vi "(Test) Chamber.vi"() -> ()   [LabVIEW 2017]
uses:
  f30135b8-ed91-49ac-be03-38adf51057fc.vi
  a24e3ecb-3937-427e-89a7-e138db600c34.vi
  c2173d89-5ae8-4599-a943-d35810f265fc.vi
  2c7cd04d-549a-457e-88ac-024da1df5a93.vi
  <vilib>/Instr/_visa.llb/VISA Configure Serial Port (Instr).vi
panel:
  out "*(타입 *) &x":string
  in  "Taget Temp":u16
  out "Data":string
  out "Write":string
  out "CRC16":string
  out "READ":string
  # "15"
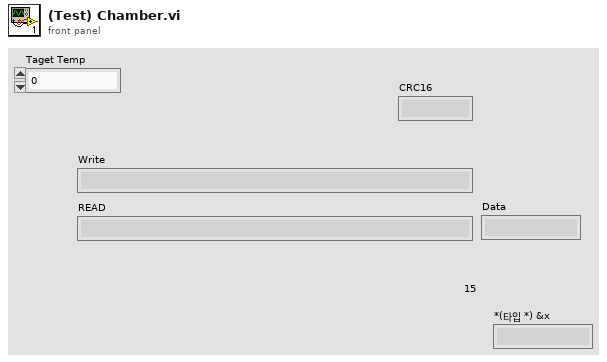
[diagram p1: front panel]
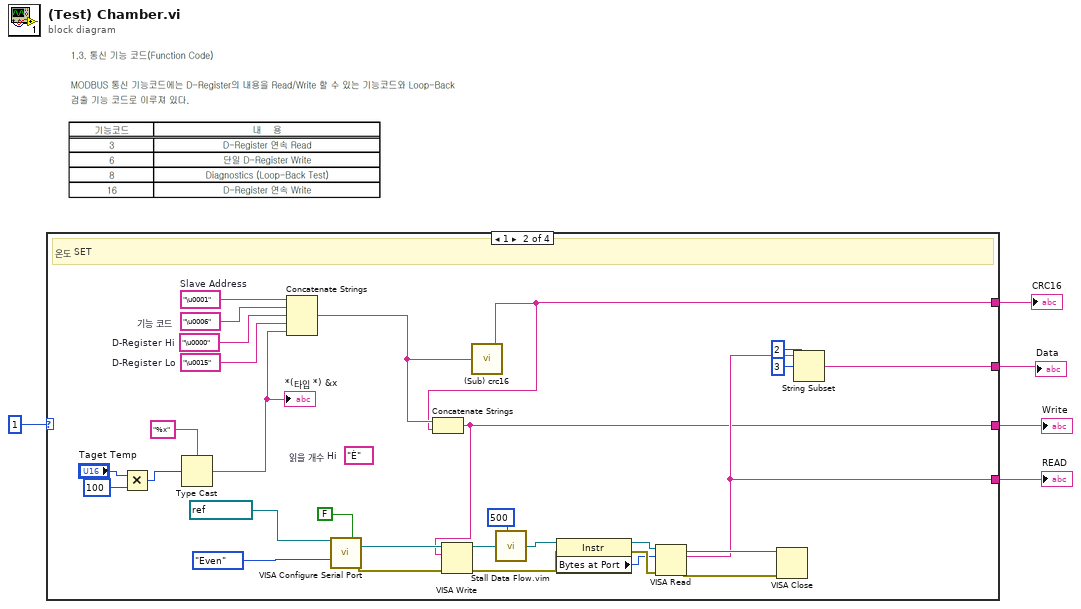
[diagram p0: block diagram]
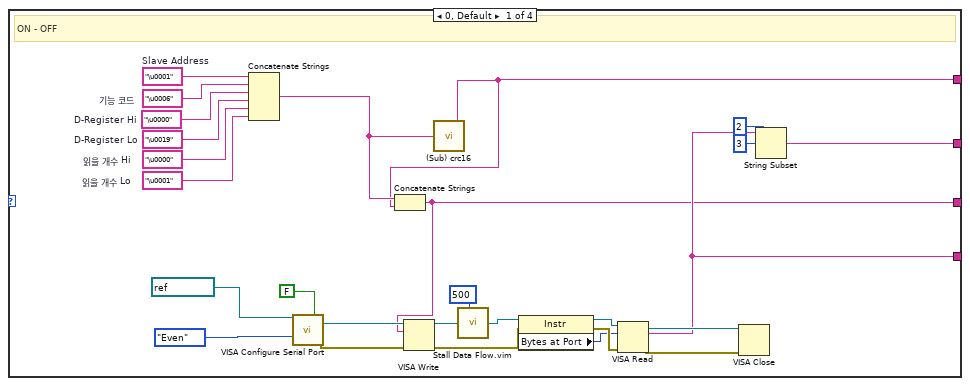
[diagram p2: hidden frame]
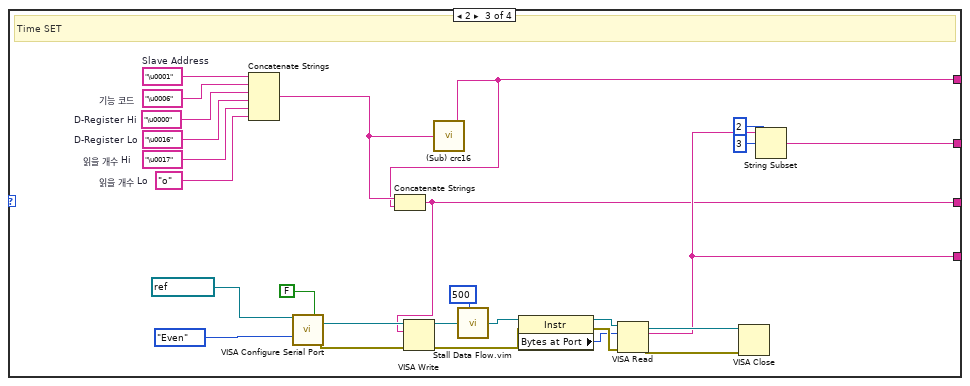
[diagram p3: hidden frame]
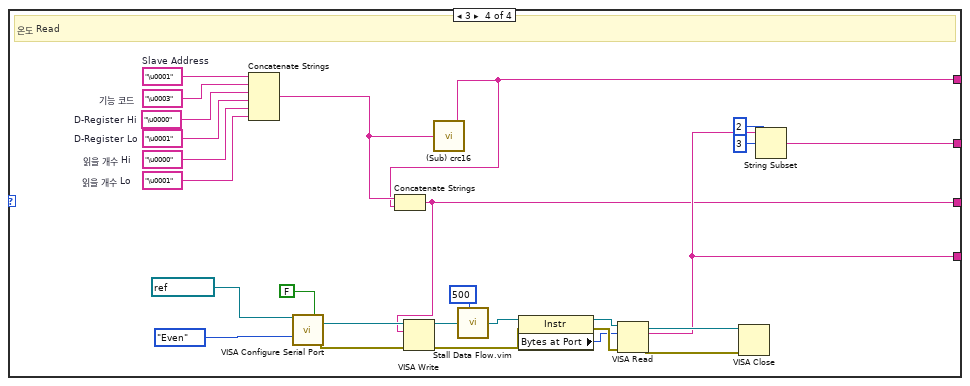
[diagram p4: hidden frame]
diagram:
  n1 = case shown="1" 1 {
    tunnel: [w9 w41 w66 w93] -> w5
    tunnel: [w8 w40 w65 w92] -> w4
    tunnel: [w7 w39 w64 w91] -> w3
    tunnel: [w6 w38 w63 w90] -> w2
    frame 0, Default {
      w10 = "\u0001"  # 읽을 개수 Lo
      w16 = "\u0000"  # 읽을 개수 Hi
      w17 = "\u0019"  # D-Register Lo
      w18 = "\u0000"  # D-Register Hi
      w19 = "\u0006"  # 기능 코드
      w20 = "\u0001"  # Slave Address
      # "ON - OFF"
      n2 = Concatenate Strings(w20, w19, w18, w17, w16, w10) -> (w15:string)
      n3 = call-poly "VISA Configure Serial Port"("VISA resource name"=refnum<visa-resource-name> "COM7", "Enable Termination\nChar (T)"=FALSE ("Enable Termination\nChar (T)"), "parity (0:none)"=enum16{"None", "Odd", "Even", "Mark", "Space"}."Even") -> ("VISA resource name out"=w32:refnum<visa-resource-name>, "error out"=w31:errorcluster)  [unwired: 11 in]
      n4 = call "(Sub) crc16.vi"("message"=w15) -> ("CRC16"=w9:string)  [unwired: 4 in]
      n5 = Concatenate Strings(w15, w9) -> (w6:string)
      n6 = VISA Write(VISA resource name=w32, write buffer=w6, error in (no error)=w31) -> (VISA resource name out=w28:refnum<visa-resource-name>, error out=w27:errorcluster)  [unwired: 1 out]
      n7 = call "Stall Data Flow.vim"("value in"=w28, "milliseconds to wait"=u32 500) -> ("value out"=w22:refnum<visa-resource-name>)  [unwired: 1 out]
      n8 = property class="Instr"(reference=w22, error in=w27) -> (reference out=w26:refnum<visa-resource-name>, error out=w25:errorcluster, "Bytes at Port"=w14:u32)
      n9 = VISA Read(VISA resource name=w26, byte count=w14, error in (no error)=w25) -> (VISA resource name out=w30:refnum<visa-resource-name>, read buffer=w7:string, error out=w29:errorcluster)  [unwired: 1 out]
      n10 = VISA Close(VISA resource name=w30, error in (no error)=w29) -> ()  [unwired: 1 out]
      n11 = String Subset(string=w7, offset (0)=3 ("오프셋(0)"), length (rest)=2 ("길이(나머지)")) -> (substring=w8:string)
    }
    frame 1 {
      (unwired) "È"  # 읽을 개수 Hi
      w47 = "\u0015"  # D-Register Lo
      w48 = "\u0000"  # D-Register Hi
      w49 = "\u0006"  # 기능 코드
      w50 = "\u0001"  # Slave Address
      # "온도 SET"
      n12 = Multiply(x="Taget Temp", y=u16 100) -> (x*y=w33:u16)
      n13 = Type Cast(type="%x" ("타입"), x=w33) -> (*(type *) &x=w36:string)
      "*(타입 *) &x" <- w36
      n14 = Concatenate Strings(w50, w49, w48, w47, w36) -> (w46:string)
      n15 = call-poly "VISA Configure Serial Port"("VISA resource name"=refnum<visa-resource-name> "COM7", "Enable Termination\nChar (T)"=FALSE ("Enable Termination\nChar (T)"), "parity (0:none)"=enum16{"None", "Odd", "Even", "Mark", "Space"}."Even") -> ("VISA resource name out"=w62:refnum<visa-resource-name>, "error out"=w61:errorcluster)  [unwired: 11 in]
      n16 = call "(Sub) crc16.vi"("message"=w46) -> ("CRC16"=w41:string)  [unwired: 4 in]
      n17 = Concatenate Strings(w46, w41) -> (w38:string)
      n18 = VISA Write(VISA resource name=w62, write buffer=w38, error in (no error)=w61) -> (VISA resource name out=w58:refnum<visa-resource-name>, error out=w57:errorcluster)  [unwired: 1 out]
      n19 = call "Stall Data Flow.vim"("value in"=w58, "milliseconds to wait"=u32 500) -> ("value out"=w52:refnum<visa-resource-name>)  [unwired: 1 out]
      n20 = property class="Instr"(reference=w52, error in=w57) -> (reference out=w56:refnum<visa-resource-name>, error out=w55:errorcluster, "Bytes at Port"=w45:u32)
      n21 = VISA Read(VISA resource name=w56, byte count=w45, error in (no error)=w55) -> (VISA resource name out=w60:refnum<visa-resource-name>, read buffer=w39:string, error out=w59:errorcluster)  [unwired: 1 out]
      n22 = VISA Close(VISA resource name=w60, error in (no error)=w59) -> ()  [unwired: 1 out]
      n23 = String Subset(string=w39, offset (0)=3 ("오프셋(0)"), length (rest)=2 ("길이(나머지)")) -> (substring=w40:string)
    }
    frame 2 {
      w67 = "o"  # 읽을 개수 Lo
      w73 = "\u0017"  # 읽을 개수 Hi
      w74 = "\u0016"  # D-Register Lo
      w75 = "\u0000"  # D-Register Hi
      w76 = "\u0006"  # 기능 코드
      w77 = "\u0001"  # Slave Address
      # "Time SET"
      n24 = Concatenate Strings(w77, w76, w75, w74, w73, w67) -> (w72:string)
      n25 = call-poly "VISA Configure Serial Port"("VISA resource name"=refnum<visa-resource-name> "COM7", "Enable Termination\nChar (T)"=FALSE ("Enable Termination\nChar (T)"), "parity (0:none)"=enum16{"None", "Odd", "Even", "Mark", "Space"}."Even") -> ("VISA resource name out"=w89:refnum<visa-resource-name>, "error out"=w88:errorcluster)  [unwired: 11 in]
      n26 = call "(Sub) crc16.vi"("message"=w72) -> ("CRC16"=w66:string)  [unwired: 4 in]
      n27 = Concatenate Strings(w72, w66) -> (w63:string)
      n28 = VISA Write(VISA resource name=w89, write buffer=w63, error in (no error)=w88) -> (VISA resource name out=w85:refnum<visa-resource-name>, error out=w84:errorcluster)  [unwired: 1 out]
      n29 = call "Stall Data Flow.vim"("value in"=w85, "milliseconds to wait"=u32 500) -> ("value out"=w79:refnum<visa-resource-name>)  [unwired: 1 out]
      n30 = property class="Instr"(reference=w79, error in=w84) -> (reference out=w83:refnum<visa-resource-name>, error out=w82:errorcluster, "Bytes at Port"=w71:u32)
      n31 = VISA Read(VISA resource name=w83, byte count=w71, error in (no error)=w82) -> (VISA resource name out=w87:refnum<visa-resource-name>, read buffer=w64:string, error out=w86:errorcluster)  [unwired: 1 out]
      n32 = VISA Close(VISA resource name=w87, error in (no error)=w86) -> ()  [unwired: 1 out]
      n33 = String Subset(string=w64, offset (0)=3 ("오프셋(0)"), length (rest)=2 ("길이(나머지)")) -> (substring=w65:string)
    }
    frame 3 {
      w94 = "\u0001"  # 읽을 개수 Lo
      w100 = "\u0000"  # 읽을 개수 Hi
      w101 = "\u0001"  # D-Register Lo
      w102 = "\u0000"  # D-Register Hi
      w103 = "\u0003"  # 기능 코드
      w104 = "\u0001"  # Slave Address
      # "온도 Read"
      n34 = Concatenate Strings(w104, w103, w102, w101, w100, w94) -> (w99:string)
      n35 = call-poly "VISA Configure Serial Port"("VISA resource name"=refnum<visa-resource-name> "COM7", "Enable Termination\nChar (T)"=FALSE ("Enable Termination\nChar (T)"), "parity (0:none)"=enum16{"None", "Odd", "Even", "Mark", "Space"}."Even") -> ("VISA resource name out"=w116:refnum<visa-resource-name>, "error out"=w115:errorcluster)  [unwired: 11 in]
      n36 = call "(Sub) crc16.vi"("message"=w99) -> ("CRC16"=w93:string)  [unwired: 4 in]
      n37 = Concatenate Strings(w99, w93) -> (w90:string)
      n38 = VISA Write(VISA resource name=w116, write buffer=w90, error in (no error)=w115) -> (VISA resource name out=w112:refnum<visa-resource-name>, error out=w111:errorcluster)  [unwired: 1 out]
      n39 = call "Stall Data Flow.vim"("value in"=w112, "milliseconds to wait"=u32 500) -> ("value out"=w106:refnum<visa-resource-name>)  [unwired: 1 out]
      n40 = property class="Instr"(reference=w106, error in=w111) -> (reference out=w110:refnum<visa-resource-name>, error out=w109:errorcluster, "Bytes at Port"=w98:u32)
      n41 = VISA Read(VISA resource name=w110, byte count=w98, error in (no error)=w109) -> (VISA resource name out=w114:refnum<visa-resource-name>, read buffer=w91:string, error out=w113:errorcluster)  [unwired: 1 out]
      n42 = VISA Close(VISA resource name=w114, error in (no error)=w113) -> ()  [unwired: 1 out]
      n43 = String Subset(string=w91, offset (0)=3 ("오프셋(0)"), length (rest)=2 ("길이(나머지)")) -> (substring=w92:string)
    }
  }
  "CRC16" <- w5
  "Data" <- w4
  "READ" <- w3
  "Write" <- w2
